vi "Insert Status for One VI.vi"(5 "error msg if NOT append error":string, 6 "VI Fail":string, 7 "append error":bool=TRUE, 8 "error in":errorcluster, 9 "VI Success":string, 10 "line no":i32, 11 "list":refnum<vi>) -> (0 "error out":errorcluster)   [LabVIEW 2020]
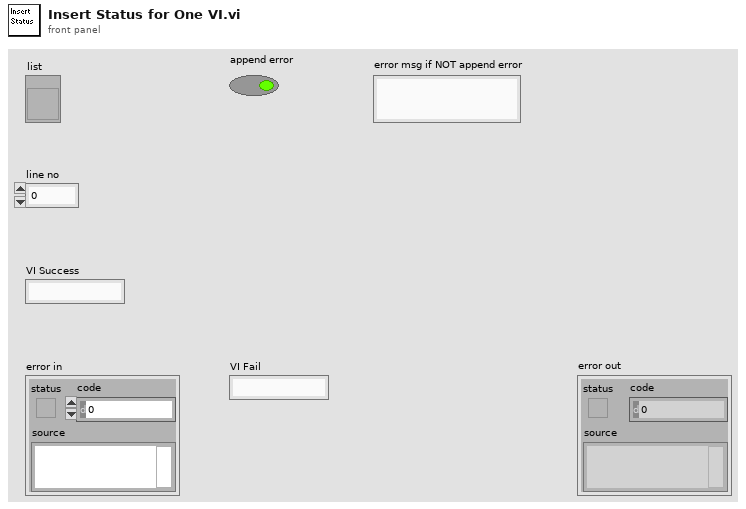
[diagram p1: front panel]
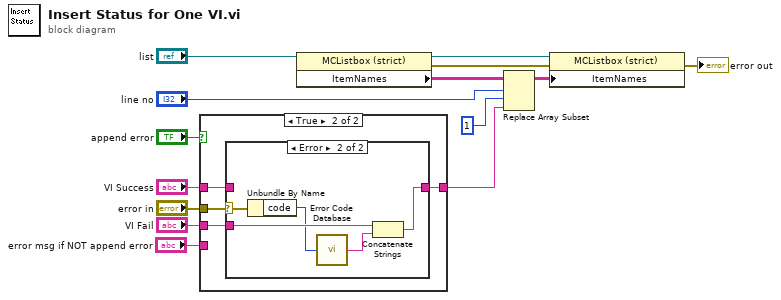
[diagram p0: block diagram]
diagram:
  n1 = case shown="True" "append error" {
    tunnel: "VI Fail" -> [_ w18]
    tunnel: "VI Success" -> [_ w17]
    tunnel: "error in" -> [_ w19]
    tunnel: [w15 w16] -> w5
    tunnel: "error msg if NOT append error" -> [w15 _]
    frame False {
    }
    frame True {
      n2 = case shown="Error" w19 {
        selector: w19 -> [_ w25]
        tunnel: [w20 w23] -> w16
        tunnel: w18 -> [_ w24]
        tunnel: w17 -> [w20 _]
        frame No Error {
        }
        frame Error {
          n3 = Unbundle By Name(w25) -> ("code"=w22:i32)
          n4 = call <vilib>:"Error Code Database.vi"("Error Code"=w22) -> ("Error Text"=w21:string)
          n5 = Concatenate Strings(w24, w21) -> (w23:string)
        }
      }
    }
  }
  n6 = property on="Property Node" class="MCListbox (strict)"(reference="list") -> (reference out=w9:refnum<vi>, error out=w14:errorcluster, "ItemNames"=w8:string[][])  [unwired: 1 in]
  n7 = Replace Array Subset(array=w8, new element=w5, index (row)="line no", index (col)=1 ("disabled index (col)")) -> (w4:string[][])
  n8 = property on="Property Node" class="MCListbox (strict)"(reference=w9, error in=w14, "ItemNames"=w4) -> (error out=→"error out":errorcluster)  [unwired: 1 out]
